vi "createListBoxLineHighlights.vi"(8 "error in (no error)":errorcluster, 10 "Listbox in":refnum<vi>, 11 "ExperimentRunner in":refnum<class "ExperimentRunner.lvclass">) -> (0 "error out":errorcluster, 2 "Listbox out":refnum<vi>, 3 "ExperimentRunner out":refnum<class "ExperimentRunner.lvclass">)   [LabVIEW 2011, in "Views.lvlib" / "ExperimentControl.lvlib" / "ExperimentRunner.lvclass"]
uses:
  ExperimentRunner.lvclass
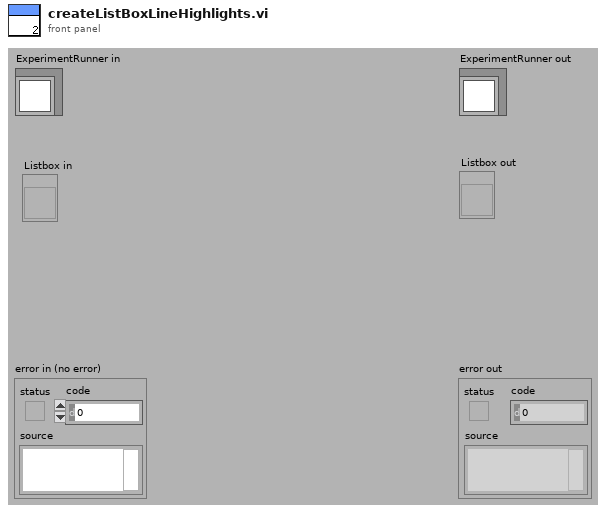
[diagram p1: front panel]
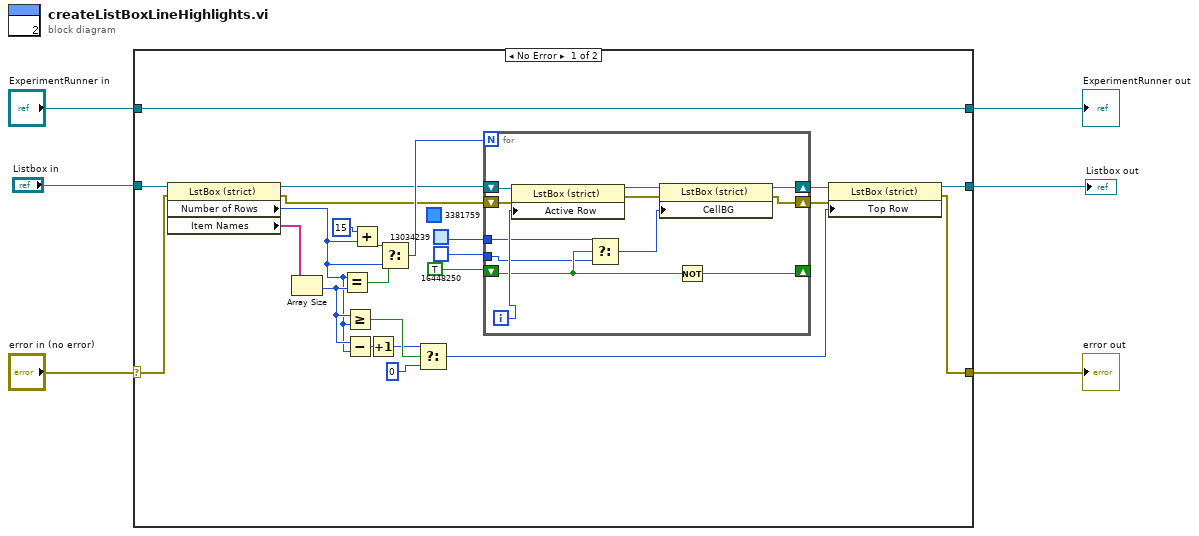
[diagram p0: block diagram]
diagram:
  n1 = case shown="No Error" "error in (no error)" {
    selector: "error in (no error)" -> [w28 w44]
    tunnel: [w16 w44] -> w5
    tunnel: [w30 w43] -> w3
    tunnel: "ExperimentRunner in" -> [w30 w43]
    tunnel: "Listbox in" -> [w29 _]
    tunnel: [w15 _] -> w1
    frame No Error {
      (unwired) u32 3381759
      n2 = property class="LstBox (strict)"(reference=w29, error in=w28) -> (reference out=w20:refnum<vi>, error out=w19:errorcluster, "Number of Rows"=w9:u32, "Item Names"=w25:string[])
      n3 = Array Size(array=w25) -> (size(s)=w10:i32)
      n4 = Equal?(x=w9, y=w10) -> (x = y?=w24:bool)
      n5 = Greater Or Equal?(x=w10, y=w9) -> (x >= y?=w14:bool)
      n6 = Subtract(x=w10, y=w9) -> (x-y=w13:u32)
      n7 = Add(x=15, y=w9) -> (x+y=w23:u32)
      n8 = Increment(x=w13) -> (x+1=w8:u32)
      n9 = Select(t=w23, s=w24, f=w9) -> (s? t:f=w21:u32)
      n10 = Select(t=w8, s=w14, f=0) -> (s? t:f=w11:u32)
      n11 = for {
        N: w21 -> [_]
        shift-right: [w32] -> w18
        shift-left: w20 -> [w42]
        shift-right: [w31] -> w17
        shift-left: w19 -> [w40]
        shift-right: [w37] -> _
        shift-left: TRUE -> [w36]
        tunnel: u32 13034239 -> [w35]
        tunnel: u32 16448250 -> [w34]
        i -> [w41]
        n12 = property class="LstBox (strict)"(reference=w42, error in=w40, "Active Row"=w41) -> (reference out=w39:refnum<vi>, error out=w38:errorcluster)
        n13 = Select(t=w35, s=w36, f=w34) -> (s? t:f=w33:u32)
        n14 = property class="LstBox (strict)"(reference=w39, error in=w38, "CellBG"=w33) -> (reference out=w32:refnum<vi>, error out=w31:errorcluster)
        n15 = Not(x=w36) -> (.not. x?=w37:bool)
      }
      n16 = property class="LstBox (strict)"(reference=w18, error in=w17, "Top Row"=w11) -> (reference out=w15:refnum<vi>, error out=w16:errorcluster)
    }
    frame Error {
    }
  }
  "error out" <- w5
  "ExperimentRunner out" <- w3
  "Listbox out" <- w1
